vi "util_get_install_path.vi"(7 "vi_reference":refnum<vi>, 8 "error in (no error)":errorcluster, 10 "zip_path":path, 11 "project_path":path) -> (0 "error out":errorcluster)   [LabVIEW 2015, in "lv-bin.lvlib" / "v1.lvlib"]
uses:
  v1.lvlib
  <vilib>/zip/NI_Unzip.lvlib
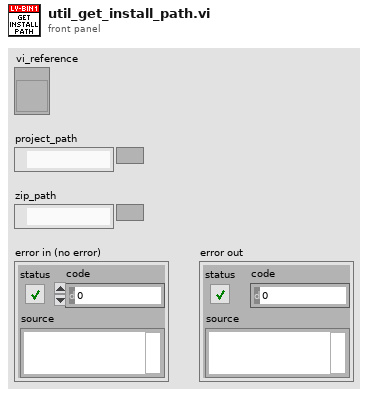
[diagram p1: front panel]
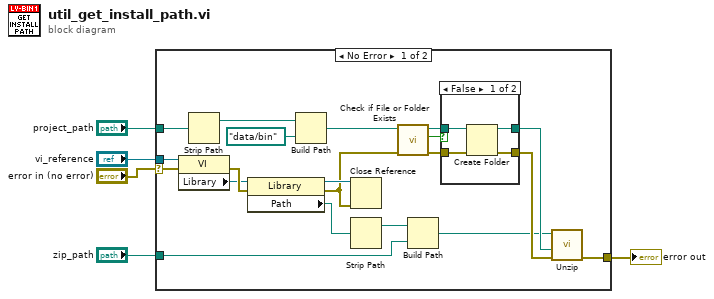
[diagram p0: block diagram]
diagram:
  n1 = case shown="No Error" "error in (no error)" {
    selector: "error in (no error)" -> [w13 w32]
    tunnel: "vi_reference" -> [w24 _]
    tunnel: [w19 w32] -> w4
    tunnel: "zip_path" -> [w12 _]
    tunnel: "project_path" -> [w7 _]
    frame No Error {
      n2 = property class="VI"(reference=w24, error in=w13) -> (error out=w14:errorcluster, "Library"=w8:refnum<vi>)  [unwired: 1 out]
      n3 = Strip Path(path=w7) -> (stripped path=w15:path)  [unwired: 1 out]
      n4 = property class="Library"(reference=w8, error in=w14) -> (reference out=w9:refnum<vi>, error out=w6:errorcluster, "Path"=w10:path)
      n5 = Build Path(base path=w15, name or relative path=path "data/bin" ("stripped path")) -> (appended path=w21:path)
      n6 = Close Reference(reference=w9, error in (no error)=w6) -> ()  [unwired: 1 out]
      n7 = Strip Path(path=w10) -> (stripped path=w11:path)  [unwired: 1 out]
      n8 = call <vilib>:"Check if File or Folder Exists.vi"("error in (no error)"=w6, "path"=w21) -> ("error out"=w20:errorcluster, "file or folder exists?"=w23:bool, "dup path"=w22:path)  [unwired: 7 in]
      n9 = Build Path(base path=w11, name or relative path=w12) -> (appended path=w17:path)
      n10 = case shown="False" w23 {
        tunnel: [w29 w30] -> w25
        tunnel: [w28 w31] -> w18
        tunnel: w20 -> [w27 w30]
        tunnel: w22 -> [w26 w31]
        frame False {
          n11 = Create Folder(path (use dialog)=w26, error in=w27) -> (created path=w28:path, error out=w29:errorcluster)  [unwired: 1 in, 1 out]
        }
        frame True {
        }
      }
      n12 = call <vilib>:"Unzip.vi"("error in (no error)"=w25, "Target directory (same as Zip file if empty)"=w18, "Zip file"=w17) -> ("error out"=w19:errorcluster)  [unwired: 6 in, 2 out]
    }
    frame Error {
    }
  }
  "error out" <- w4
